vi "RelayClose_L.vi"(0 "datain":string[](array[string])=["备注", "负载通道", "负载地址", "延时时间", "output max", "output min", "量测类型", "待测物板号"], 5 "HW CH Number":i32=4, 7 "Setup":string="1") -> (4 "REPORT INDECATE":string[][](array[string])=[["微安测试", "", "", "", ""], ["微安量测", "4", "0.000", "0.1", "NG"], ["微安量测", "4", "0.000", "0.1", "NG"], ["微安量测", "4", "0.000", "0.1", "NG"], ["微安量测", "4", "0.000", "0.1", "NG"]], 6 "ROW HEAD":string[](array[string]), 8 "PF":string[](array[string]), 10 "testData":string[](array[string]), 14 "数组":bool[](array[boolean]), 15 "Array":string[](array[string]))   [LabVIEW 2018]
uses:
  Subvi/Global.vi
panel:
  out "L":string
  out "H":string
  out "测试板数":i32=4
  # "Ext.Name =Open_AC230;\nAddress =0;\nDelay Time =2000;\nMAX.Spec =*;\nMin.Spec =*;\nTest Type =4;\nRelayH_8Bit =7,0,0,7;\nRelayL_8Bit =0,0,0,0;\nStandby Application =;\nStart board number =1;#"
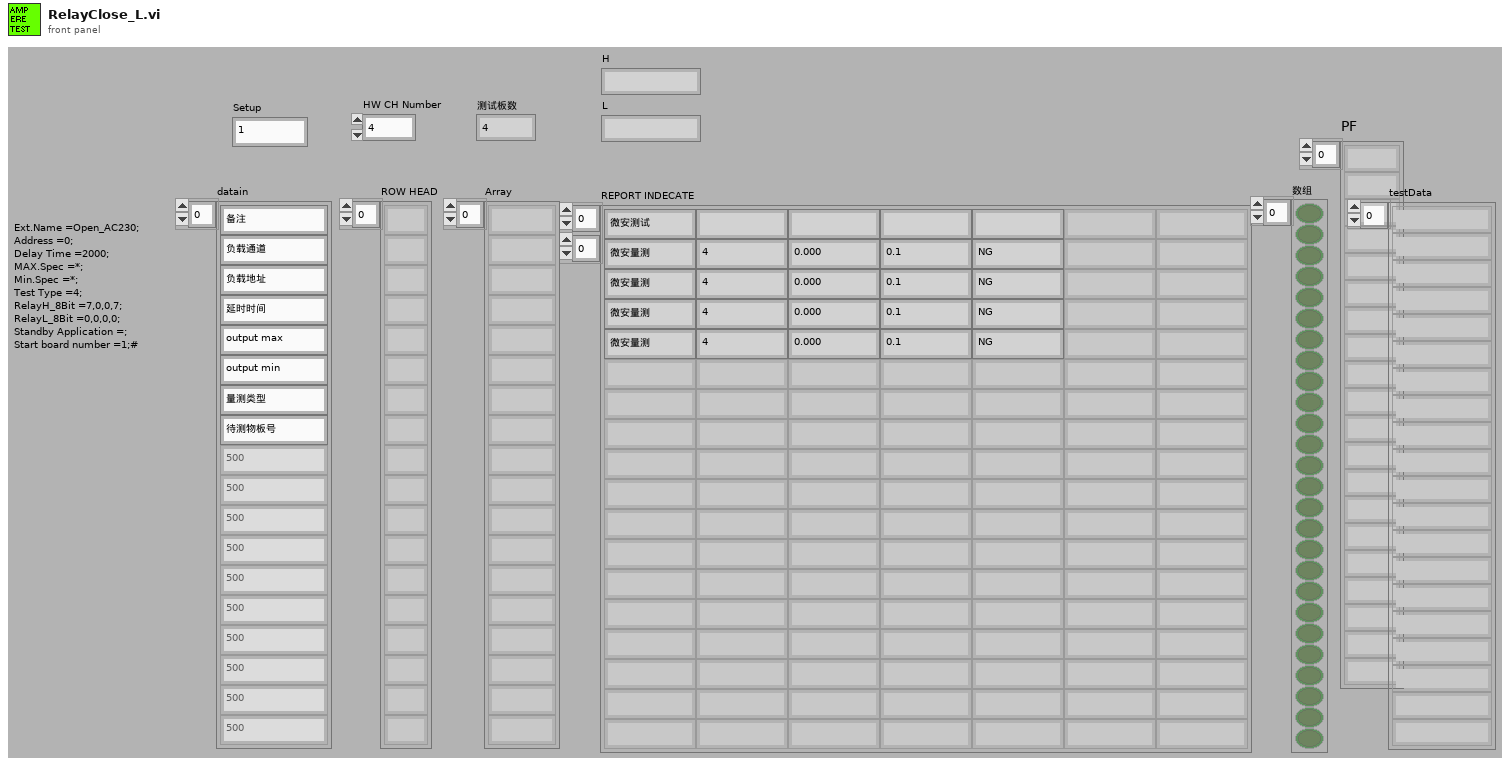
[diagram p1: front panel]
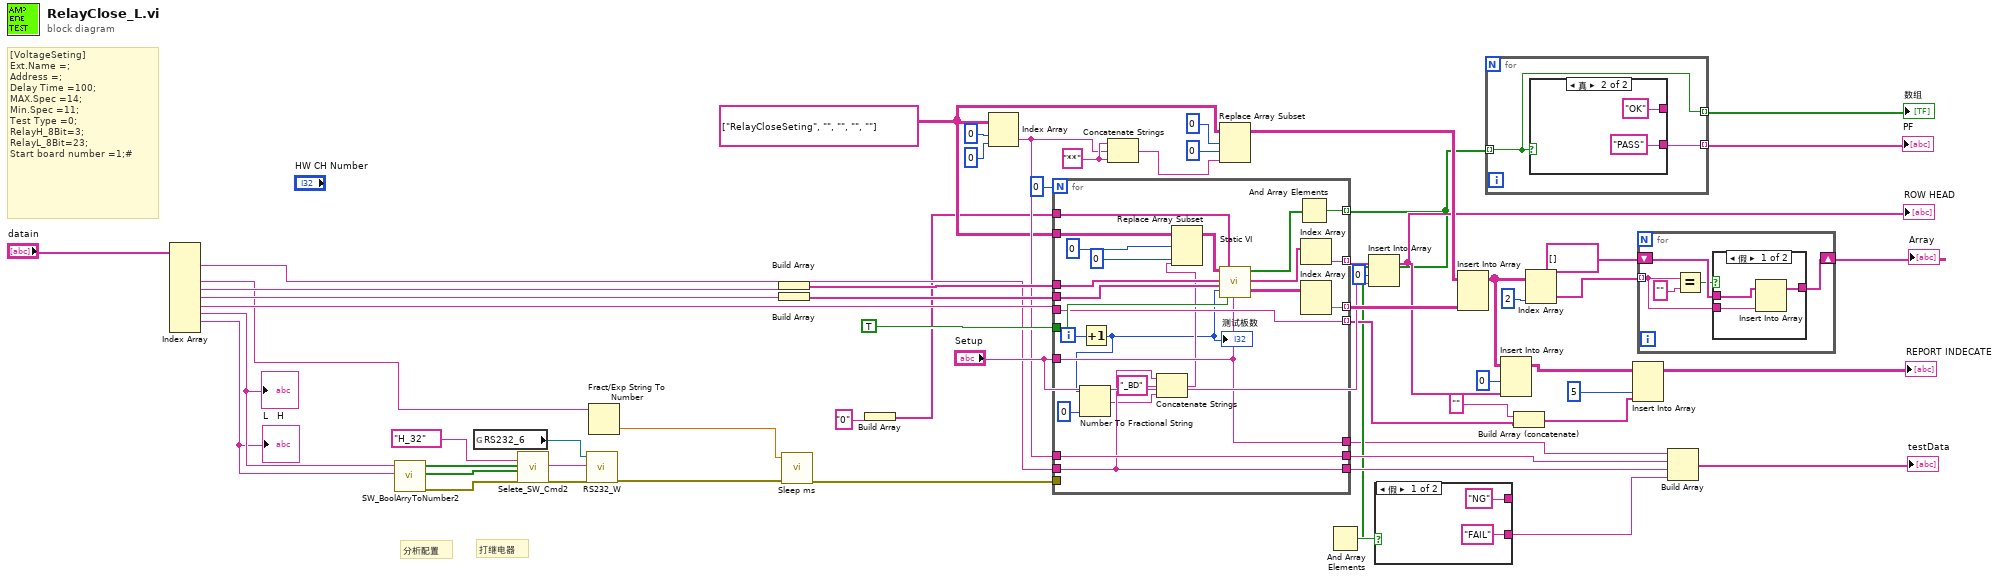
[diagram p0: block diagram]
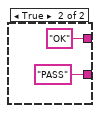
[diagram p2: hidden frame]
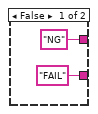
[diagram p3: hidden frame]
diagram:
  w17 = string[][] [["RelayCloseSeting", "", "", "", ""]]
  w51 = "**" ("字符串")
  # "分析配置"
  # "打继电器"
  # "[VoltageSeting]\nExt.Name =;\nAddress =;\nDelay Time =100;\nMAX.Spec =14;\nMin.Spec =11;\nTest Type =0;\nRelayH_8Bit=3;\nRelayL_8Bit=23;\nStart board number =1;#"
  n1 = Index Array(array="datain") -> (element #1=w18:string, element #3=w8:string, element #4=w47:string, element #5=w46:string, element #6=w34:string, element #7=w6:string, element #8=w5:string)  [unwired: 9 in, 2 out]
  "H" <- w6
  "L" <- w5
  n2 = call "SW_BoolArryToNumber2.vi"("L32 INUPT"=w5, "H32 INUPT"=w6) -> ("error out"=w9:errorcluster, "L_32"=w10:bool[], "H_32"=w11:bool[])  [unwired: 6 in, 1 out]
  n3 = global read "Global.vi" "RS232_6"() -> (w1:refnum<visa-resource-name>)
  n4 = call "Selete_SW_Cmd2.vi"("组合框"="H_32", "H_32"=w11, "L_32"=w10, "error in (no error)"=w9) -> ("ColseStr"=w2:string, "error out"=w4:errorcluster)  [unwired: 12 in, 2 out]
  n5 = call "RS232_W.vi"("error in (no error)"=w4, "CMD"=w2, "VISA资源名称"=w1) -> ("error out"=w3:errorcluster)  [unwired: 6 in, 2 out]
  n6 = Fract/Exp String To Number(string=w8) -> (number=w13:dbl)  [unwired: 3 in, 1 out]
  n7 = Build Array(w47) -> (w45:string[])
  n8 = Build Array(w46) -> (w44:string[])
  n9 = call "Sleep ms.vi"("error in (no error)"=w3, "等待时间（毫秒）"=w13) -> ("error out"=w7:errorcluster)  [unwired: 9 in]
  n10 = Build Array("0") -> (w15:string[])
  n11 = Index Array(array=w17, index (row)=0 ("索引 (行)"), index (col)=0 ("禁用的索引 (列)")) -> (element=w27:string)
  n12 = for {
    N: 0 -> [_]
    tunnel: w15 -> [w83]
    tunnel: w45 -> [w82]
    tunnel: w44 -> [w81]
    tunnel: "Setup" -> [w71]
    tunnel: TRUE -> [w79]
    tunnel: [w78] -> w23 mode=indexing
    tunnel: [w76] -> w40 mode=indexing
    tunnel: [w74] -> w41 mode=indexing
    tunnel: w34 -> [w73]
    tunnel: [w73] -> w30 mode=indexing
    tunnel: w27 -> [w72]
    tunnel: [w72] -> w26
    tunnel: w18 -> [w63]
    tunnel: [w63] -> w25
    tunnel: [w71] -> w20
    tunnel: w17 -> [w69]
    tunnel: w7 -> [_]
    i -> [w66]
    n13 = Increment(x=w66) -> (x+1=w60:i32)
    "测试板数" <- w60
    n14 = Number To Fractional String(number=w60, precision (6)=i16 0 ("精度(6)")) -> (F-format string=w62:string)  [unwired: 2 in]
    n15 = Concatenate Strings(w63, "_BD" ("字符串"), w62) -> (w61:string)
    n16 = Replace Array Subset(array=w69, new element=w61, index (row)=0 ("索引 (行)"), index (col)=0 ("禁用的索引 (列)")) -> (w68:string[][])
    n17 = call "Static VI.vi"("添加的数组"=w68, "Max"=w82, "Min"=w81, "板数"=w60, "INPUTSTRING"=w83, "是否为字符串对比"=w79, "SQ"=w71) -> ("P/F"=w80:bool[], "SQ out"=w77:string[], "arrauy out"=w75:string[][])  [unwired: 9 in, 1 out]
    n18 = And Array Elements(Boolean array=w80) -> (logical AND=w78:bool)
    n19 = Index Array(array=w77) -> (element=w76:string)  [unwired: 1 in]
    n20 = Index Array(array=w75) -> (element=w74:string[])  [unwired: 2 in]
  }
  n21 = Concatenate Strings(w51, w27, w51) -> (w48:string)
  n22 = Replace Array Subset(array=w17, new element=w48, index (row)=0 ("索引 (行)"), index (col)=0 ("禁用的索引 (列)")) -> (w42:string[][])
  n23 = And Array Elements(Boolean array=w23) -> (logical AND=w24:bool)
  n24 = Insert Into Array(array=w40, index=0 ("索引"), new element="Setup") -> (w36:string[])
  "ROW HEAD" <- w36
  n25 = case shown="假" w24 {
    tunnel: ["NG" "OK"] -> _
    tunnel: ["FAIL" "PASS"] -> w22
    frame False {
    }
    frame True {
    }
  }
  n26 = Insert Into Array ("数组插入")(array=w42, new element=w41) -> (w37:string[][])  [unwired: 2 in]
  n27 = for {
    tunnel: w23 -> [w88] mode=indexing
    tunnel: [w89] -> w55 mode=indexing
    tunnel: [w88] -> w19 mode=indexing
    n28 = case shown="真" w88 {
      tunnel: ["NG" "OK"] -> _
      tunnel: ["FAIL" "PASS"] -> w89
      frame False {
      }
      frame True {
      }
    }
  }
  "PF" <- w55
  "数组" <- w19
  n29 = Insert Into Array(array=w37, index (col)=0 ("禁用的索引 (列)"), new element=w36) -> (w32:string[][])  [unwired: 1 in]
  n30 = Build Array (concatenate)("" ("字符串"), w30) -> (w28:string[])
  n31 = Index Array(array=w37, index (col)=2 ("禁用的索引 (列)")) -> (element=w57:string[])  [unwired: 1 in]
  n32 = Insert Into Array(array=w32, index (col)=5 ("禁用的索引 (列)"), new element=w28) -> (→"REPORT INDECATE":string[][])  [unwired: 1 in]
  n33 = for {
    tunnel: w57 -> [w94] mode=indexing
    shift-right: [w95] -> w56
    shift-left: string[] [] ("Array") -> [w98]
    n34 = Equal?(x=w94, y="") -> (x = y?=w96:bool)
    n35 = case shown="假" w96 {
      tunnel: w98 -> [w101 w102]
      tunnel: [w100 w102] -> w95
      tunnel: w94 -> [w99 _]
      frame False {
        n36 = Insert Into Array(array=w101, new element=w99) -> (w100:string[])  [unwired: 1 in]
      }
      frame True {
      }
    }
  }
  "Array" <- w56
  n37 = Build Array(w20, w26, w25, w22) -> (→"testData":string[])
